vi "ExcelReportSubVI.vi"(6 "start (0, 0)":cluster{"row":i32, "column":i32}, 8 "error in (no error)":errorcluster, 9 "Yazılacak Parametre":string, 10 "Test İn":string[][](table) caption="Table İn", 11 "report in":refnum<class "NI_report.lvclass">) -> (0 "error out":errorcluster, 2 "Table out":string[][](table), 3 "report out":refnum<class "NI_report.lvclass">)   [LabVIEW 2021]
uses:
  <vilib>/Utility/NIReport.llb/NI_report.lvclass
  <vilib>/addons/_office/excel.llb/Excel Easy Table (str).vi
  <vilib>/addons/_office/NI_ReportGenerationToolkit.lvlib
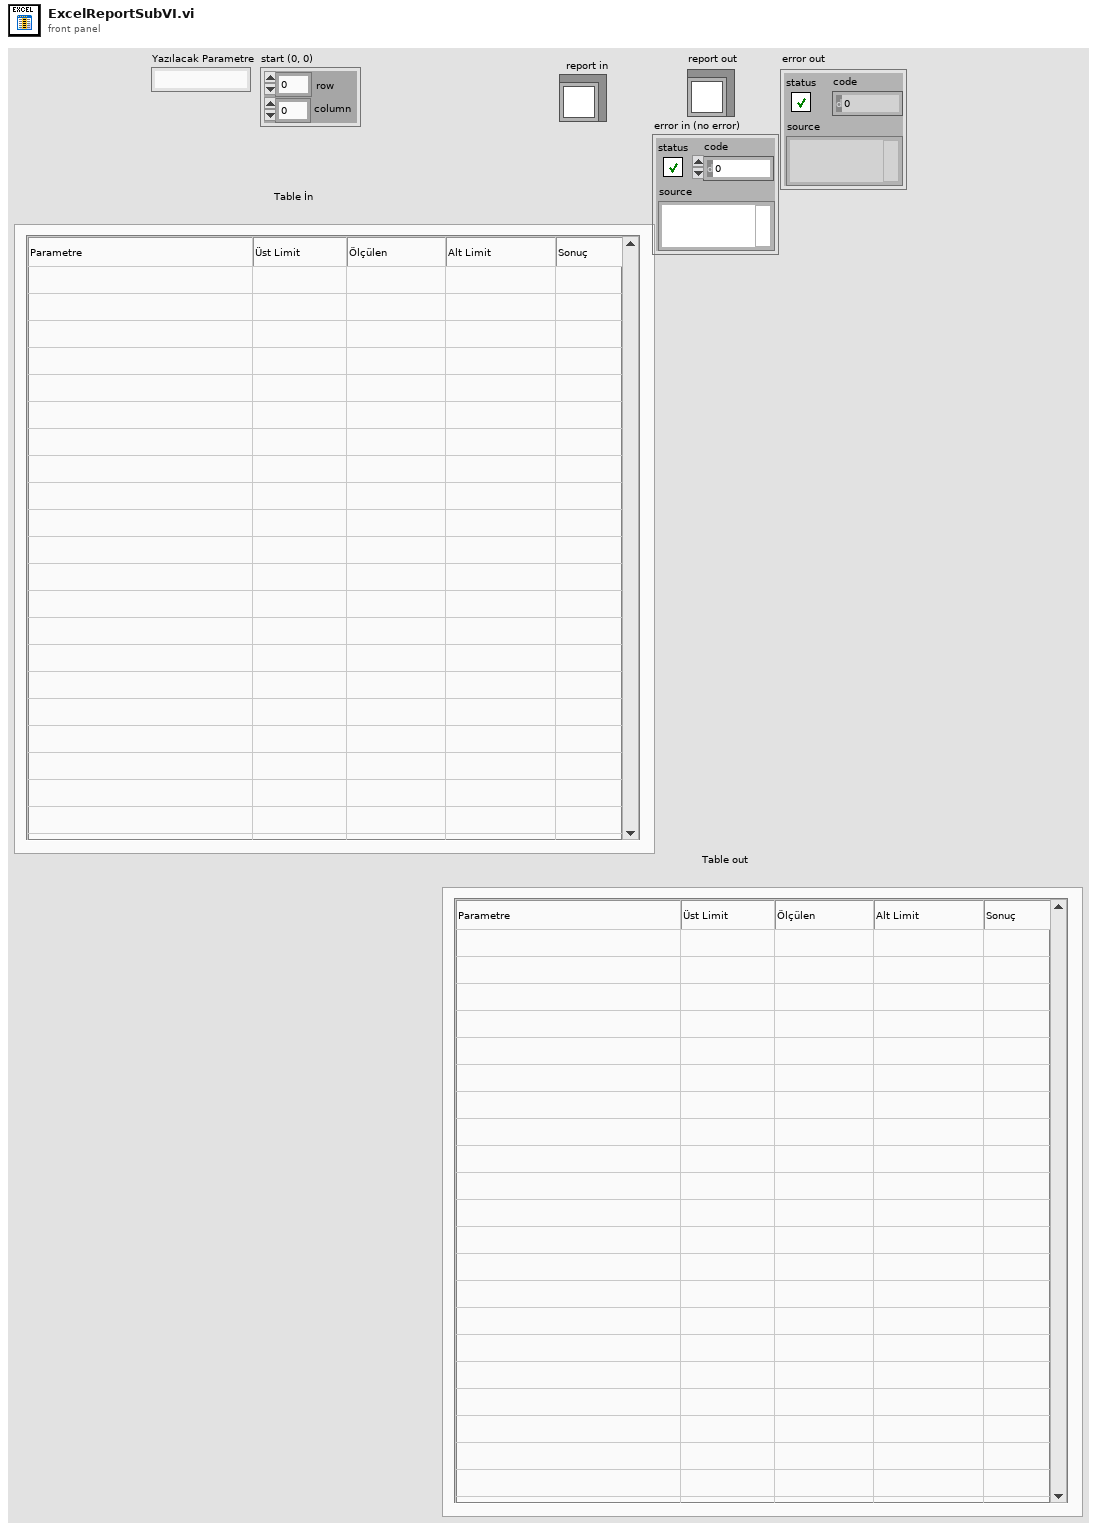
[diagram p1: front panel]
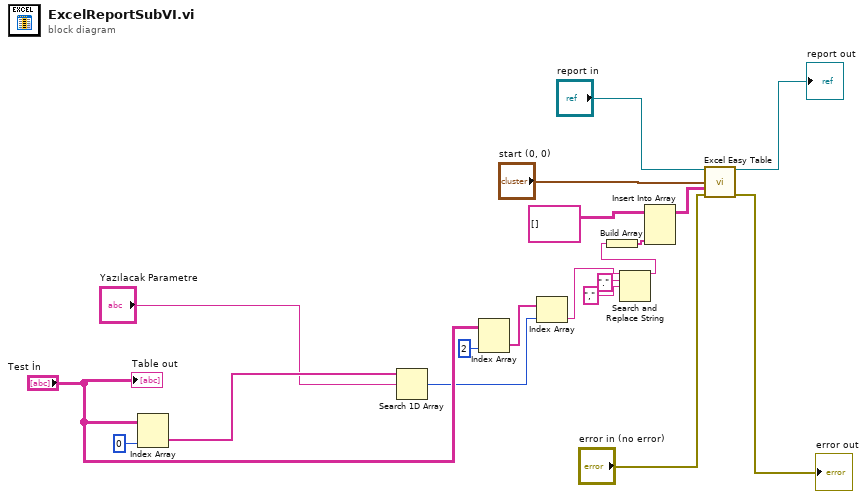
[diagram p0: block diagram]
diagram:
  n1 = Index Array(array="Test İn", index (col)=0 ("disabled index (col)")) -> (element=w13:string[])  [unwired: 1 in]
  n2 = Search 1D Array(1D array=w13, element="Yazılacak Parametre") -> (index of element=w8:i32)  [unwired: 1 in]
  n3 = Index Array(array="Test İn", index (col)=2 ("disabled index (col)")) -> (element=w9:string[])  [unwired: 1 in]
  n4 = Index Array(array=w9, index=w8) -> (element=w7:string)
  n5 = Search and Replace String(input string=w7, search string=".", replace string="," ("replace string (\"\")")) -> (result string=w14:string)  [unwired: 5 in, 3 out]
  n6 = Build Array(w14) -> (w17:string[])
  n7 = Insert Into Array(array=string[][] [] ("text data"), new element=w17) -> (w6:string[][])  [unwired: 2 in]
  n8 = call-poly <vilib>:"Excel Easy Table.vi"("report in"="report in", "start (0, 0)"="start (0, 0)", "text data"=w6, "error in (no error)"="error in (no error)") -> ("report out"=→"report out":refnum<class "NI_report.lvclass">, "error out"=→"error out":errorcluster)  [unwired: 7 in, 3 out]
  "Table out" <- "Test İn"
